vi "misc-global.vi"(1 "misc in":cluster{"Colormaps":u32[][]}, 2 "command":string) -> (0 "misc out":cluster{"Colormaps":u32[][]})   [LabVIEW 2015]
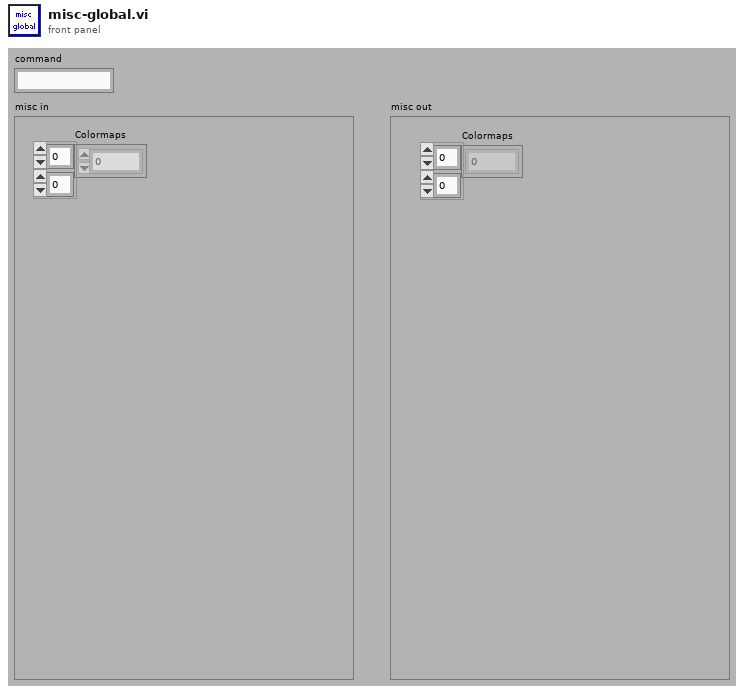
[diagram p1: front panel]
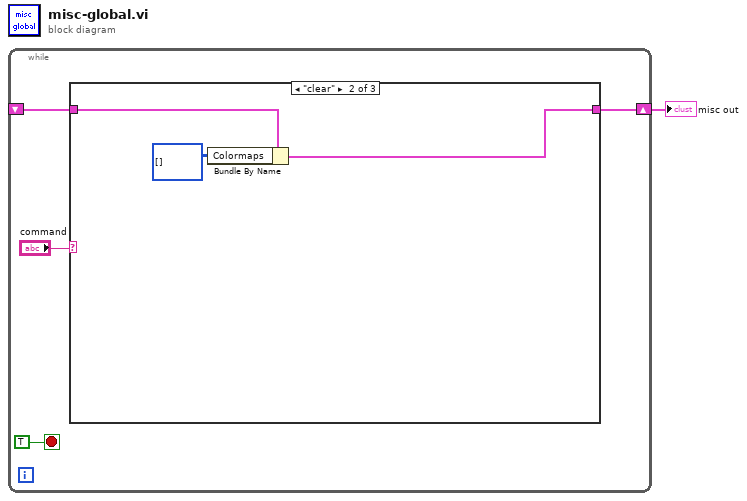
[diagram p0: block diagram]
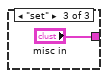
[diagram p3: hidden frame]
diagram:
  n1 = while {
    shift-right: [w3] -> w1
    shift-left: _ -> [w2]
    stop <- TRUE stop-if-true
    n2 = case shown="\"clear\"" "command" {
      tunnel: [w6 w8 "misc in"] -> w3
      tunnel: w2 -> [w6 w9 _]
      frame "get", Default {
      }
      frame "clear" {
        n3 = Bundle By Name(cluster=w9, "Colormaps"=u32[][] []) -> (w8:cluster{"Colormaps":u32[][]})
      }
      frame "set" {
      }
    }
  }
  "misc out" <- w1
